vi "Rename Log File.vi"(8 "error in":errorcluster, 10 "file name":string, 11 "log file in":T1 format="%.0x") -> (0 "error out":errorcluster, 3 "log file out":T1 format="%.0x")   [LabVIEW 2027, in "Embedded Data Logger Scripting.lvlib"]
uses:
  Embedded Data Logger Scripting.lvlib
  <vilib>/NI VeriStand/Custom Device API/Custom Device Item Ref.ctl
  <vilib>/NI VeriStand/Custom Device API/Custom Device API.lvlib
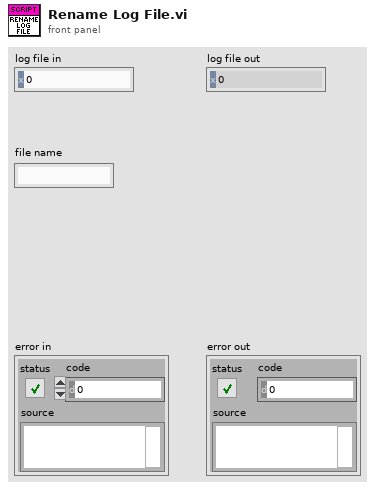
[diagram p1: front panel]
types:
  T1 = typedef "Custom Device API.lvlib/Custom Device Item Ref.ctl" = u64
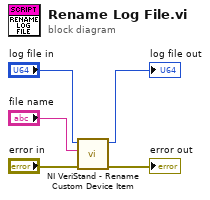
[diagram p0: block diagram]
diagram:
  n1 = call <vilib>:"NI VeriStand - Rename Custom Device Item.vi"("error in (no error)"="error in", "New Name"="file name", "Item Ref in"="log file in") -> ("error out"=→"error out":errorcluster, "Item Ref out"=→"log file out":T1)  [unwired: 6 in, 1 out]
